vi "Generate grid series (SubVI).vi"(6 "min separation":i32, 7 "separation step":i32, 8 "Move one spot":bool, 9 "Number of steps":dbl, 10 "Spots y":i32, 11 "Spots x":i32) -> (1 "Array 2":i32[][](array[numeric]), 2 "Array":i32[][](array[numeric]), 3 "Numeric out":i32, 4 "Z":i32[][](array[numeric]), 5 "A":i32[][](array[numeric]))   [LabVIEW 2011]
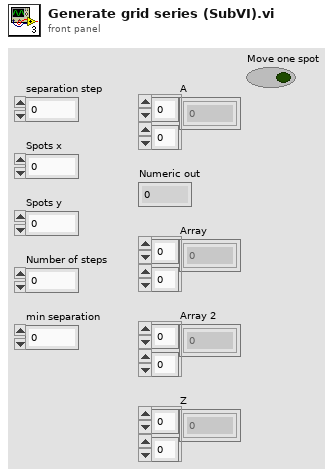
[diagram p1: front panel]
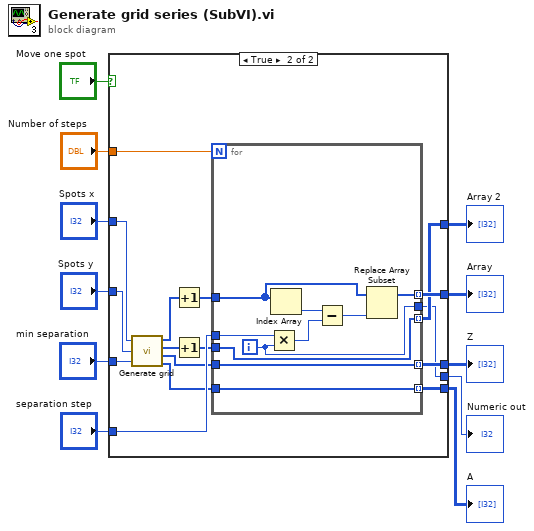
[diagram p0: block diagram]
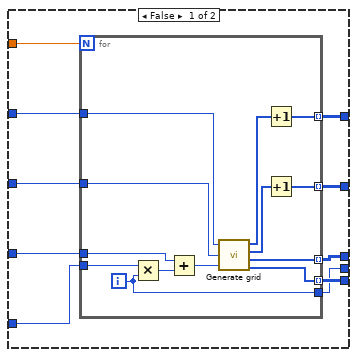
[diagram p2: hidden frame]
diagram:
  n1 = case shown="True" "Move one spot" {
    tunnel: [w21 w39] -> w11
    tunnel: [w20 w41] -> w10
    tunnel: [w19 w45] -> w9
    tunnel: [w18 w43] -> w8
    tunnel: [w17 w37] -> w7
    tunnel: "Spots y" -> [w16 w50]
    tunnel: "Spots x" -> [w15 w49]
    tunnel: "separation step" -> [w14 w46]
    tunnel: "min separation" -> [w13 w48]
    tunnel: "Number of steps" -> [w12 w38]
    frame False {
      n2 = for {
        N: w12 -> [_]
        tunnel: w13 -> [w34]
        tunnel: w14 -> [w31]
        tunnel: w15 -> [w30]
        tunnel: w16 -> [w29]
        tunnel: [w28] -> w17
        tunnel: [w23] -> w18 mode=indexing
        tunnel: [w22] -> w19 mode=indexing
        tunnel: [w25] -> w20 mode=indexing
        tunnel: [w24] -> w21 mode=indexing
        i -> [w28]
        n3 = Multiply(x=w31, y=w28) -> (x*y=w32:i32)
        n4 = Add(x=w34, y=w32) -> (x+y=w33:i32)
        n5 = call "Generate grid.vi"("Spots x"=w30, "Spots y"=w29, "Grid spacing"=w33) -> ("X"=w27:i32[], "Y"=w26:i32[], "Z"=w25:i32[], "I"=w24:i32[])
        n6 = Increment(x=w27) -> (x+1=w23:i32[])
        n7 = Increment(x=w26) -> (x+1=w22:i32[])
      }
    }
    frame True {
      n8 = call "Generate grid.vi"("Spots x"=w49, "Spots y"=w50, "Grid spacing"=w48) -> ("X"=w47:i32[], "Y"=w44:i32[], "Z"=w42:i32[], "I"=w40:i32[])
      n9 = Increment(x=w47) -> (x+1=w36:i32[])
      n10 = Increment(x=w44) -> (x+1=w35:i32[])
      n11 = for {
        N: w38 -> [_]
        tunnel: w36 -> [w60]
        tunnel: w46 -> [w53]
        tunnel: [w57] -> w45 mode=indexing
        tunnel: w35 -> [w56]
        tunnel: [w56] -> w43 mode=indexing
        tunnel: w42 -> [w55]
        tunnel: [w55] -> w41 mode=indexing
        tunnel: w40 -> [w54]
        tunnel: [w54] -> w39 mode=indexing
        tunnel: [w51] -> w37
        i -> [w51]
        n12 = Multiply(x=w53, y=w51) -> (x*y=w52:i32)
        n13 = Index Array(array=w60) -> (element=w59:i32)  [unwired: 1 in]
        n14 = Subtract(x=w59, y=w52) -> (x-y=w58:i32)
        n15 = Replace Array Subset(array=w60, new element=w58) -> (w57:i32[])  [unwired: 1 in]
      }
    }
  }
  "A" <- w11
  "Z" <- w10
  "Array" <- w9
  "Array 2" <- w8
  "Numeric out" <- w7
